vi "CompRun.vi"(0 "Initial Soak":T1(ring)=enum."5 mins", 1 "Nominal":dbl=1.0 min=0.0 max=1000.0 format="%.4f", 2 "Frequency Channel":enum16{"Channel 1", "Channel 2", "Channel 3"}(ring), 3 "Tolerence":dbl=0.01 min=0.001 max=100.0 format="%.2f", 4 "Dmm Readings":i8=5 min=0 max=5 step=1, 5 "Step Soak":T1(ring)=enum."5 mins", 6 "Gate Time":T2(ring)=enum."1.0 second", 7 "HP Switcher Address":cluster{"GPIB":u8, "Address":u8}={"GPIB"=1, "Address"=6} {"Address" min=1 max=31; "GPIB" min=1 max=5}, 8 "Temperature Array":dbl[](array[numeric]), 9 "Final Soak":T1(ring)=enum."5 mins", 11 "Slew Rate":enum16{"0.5", "1", "2"}(ring)=enum."1", 12 "V inj Min":dbl min=0.0 max=20.0 format="%.4f", 14 "Vinj Max":dbl=6.0 min=-6.0 max=20.0 format="%.4f", 15 "Chamber Address":cluster{"GPIB #":u8, "Address":u8}={"GPIB #"=0, "Address"=28}) -> ()   [LabVIEW 2024]
panel:
  out "Output File":path
  in  "DC_SN(s)":string[](array[string])
  in  "WorkOrder":string
  in  "NumberOfUnits":i32
  in  "Output Terminals(+6 V:0)":u16(ring) items=["+6 V output", "+25 V output", "-25 V output"]
  in  "Frequency Counter Address":i16=3 max=31
  out "Measured Frequency":dbl[](array[numeric]) format="%.6f"
  out "Pullability":dbl[](array[numeric]) format="%.6f"
  out "Error":dbl[](array[numeric]) format="%.2f"
  out "Iteration Successful":bool[](array[boolean])
  out "V_inject":dbl[](array[numeric]) format="%.6f"
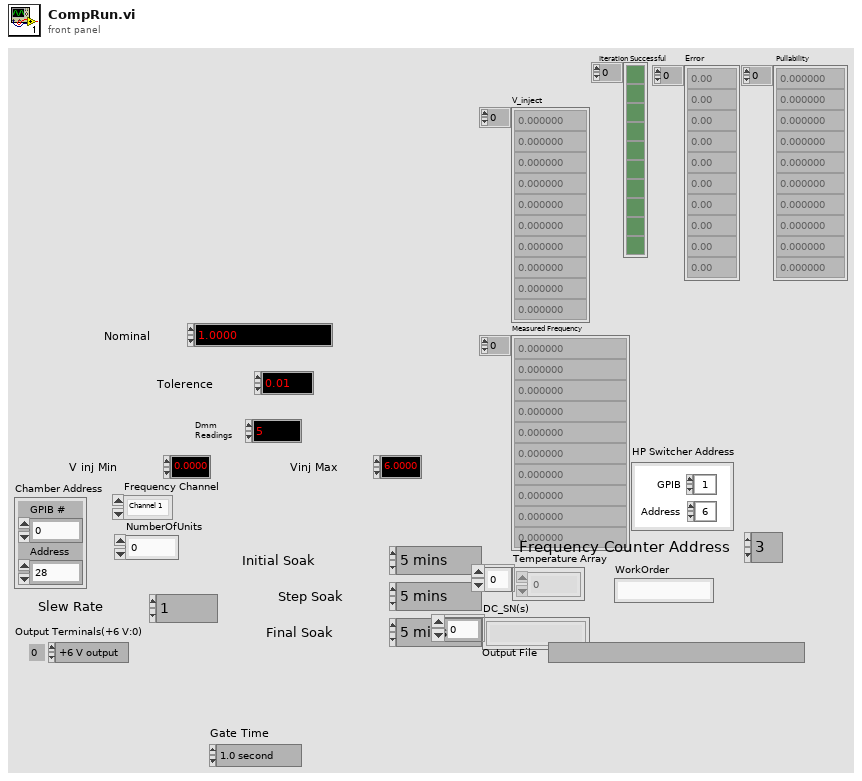
[diagram p1: front panel]
types:
  T1 = enum16{"1 min", "5 mins", "10 mins", "20 mins", "30 mins", "40 mins", "50 mins", "1 hour", "2 hours", "3 hours"}
  T2 = enum16{"0.1 second", "1.0 second", "10.0 second"}
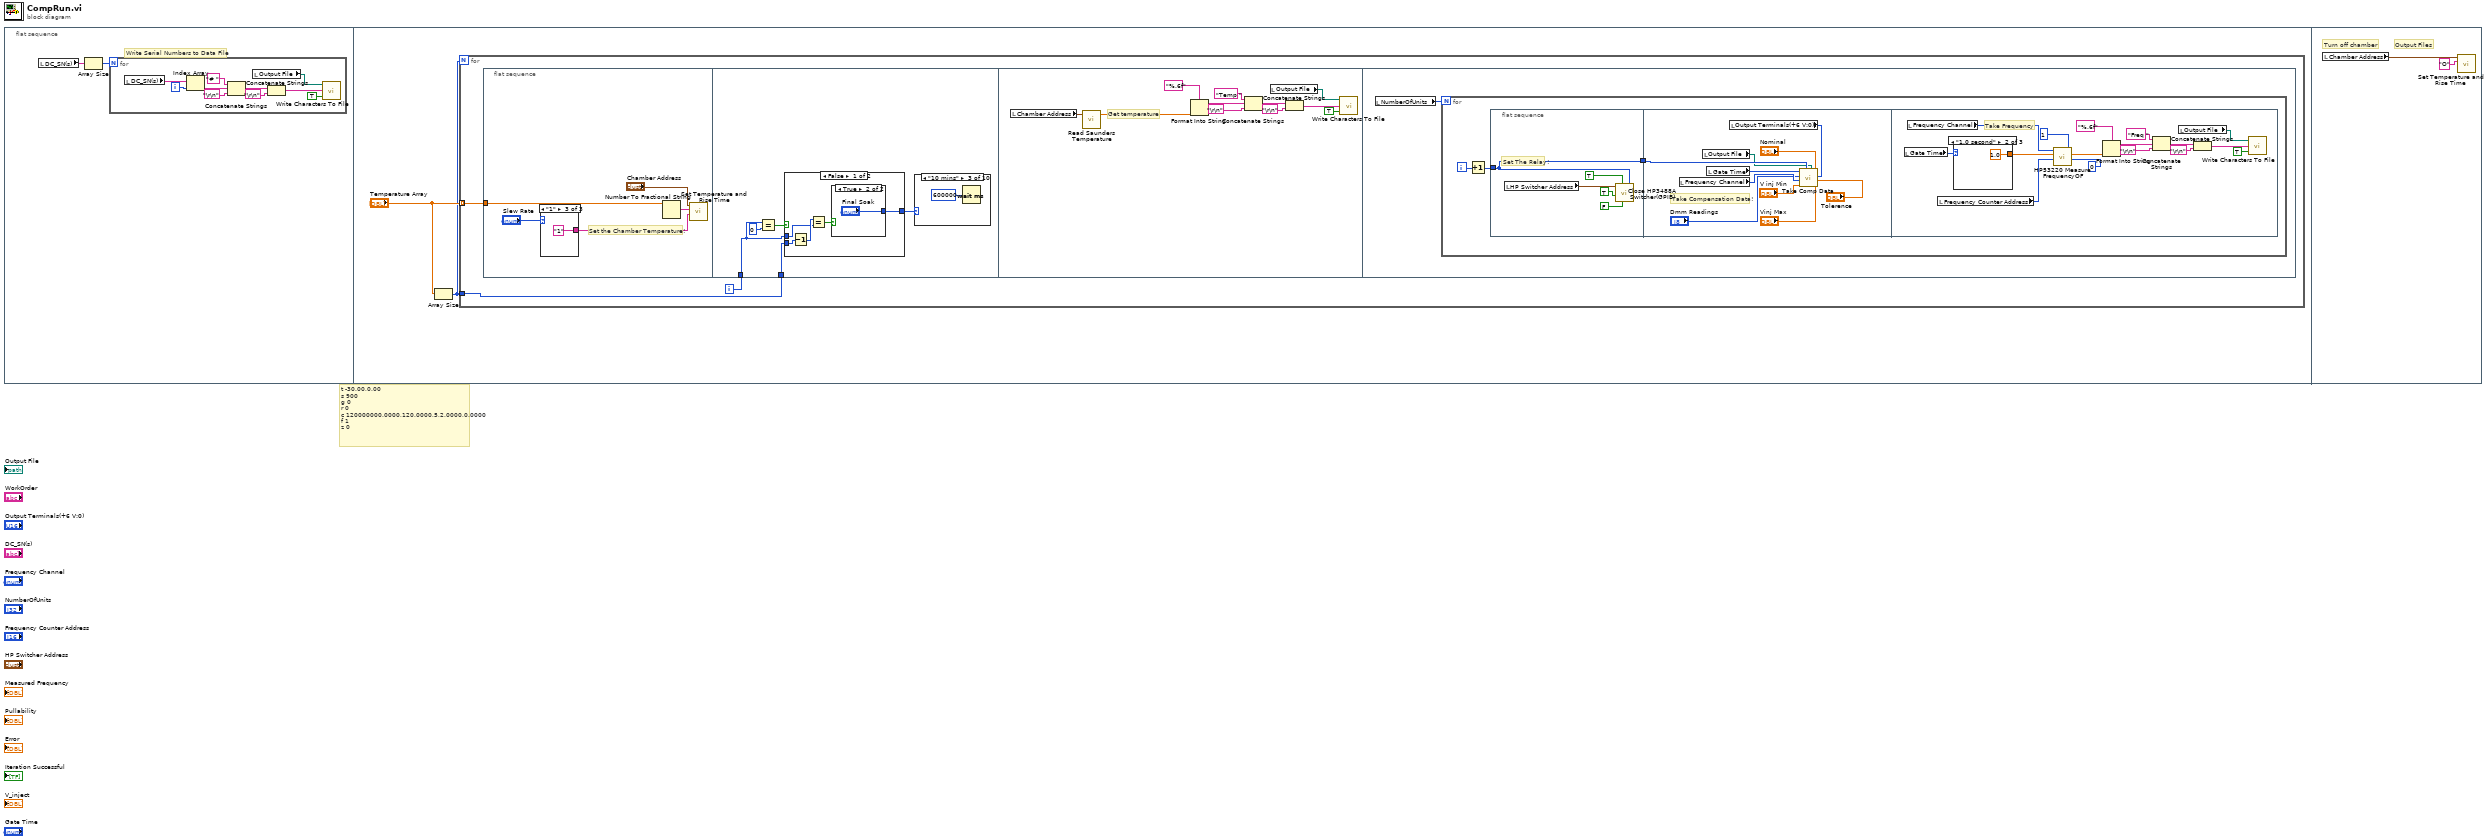
[diagram p0: block diagram]
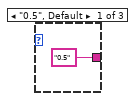
[diagram p2: hidden frame]
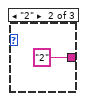
[diagram p3: hidden frame]
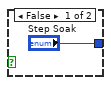
[diagram p4: hidden frame]
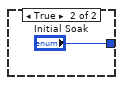
[diagram p5: hidden frame]
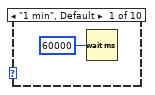
[diagram p6: hidden frame]
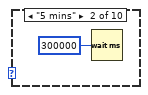
[diagram p7: hidden frame]
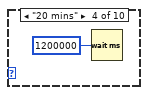
[diagram p8: hidden frame]
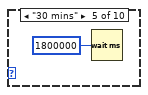
[diagram p9: hidden frame]
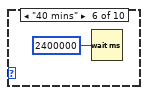
[diagram p10: hidden frame]
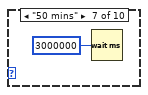
[diagram p11: hidden frame]
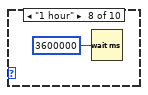
[diagram p12: hidden frame]
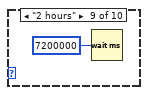
[diagram p13: hidden frame]
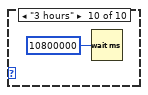
[diagram p14: hidden frame]
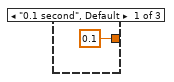
[diagram p15: hidden frame]
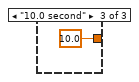
[diagram p16: hidden frame]
diagram:
  # "t -30.00,0.00\ns 900\ng 0\nr 0\nc 120000000.0000,120.0000,5,2.0000,0.0000\nf 1\nz 0"
  n1 = flat-sequence {
    frame #0 {
      # "Write Serial Numbers to Data File"
      n2 = local read "DC_SN(s)"() -> (w1:string[])
      n3 = Array Size(array=w1) -> (size(s)=w2:i32)
      n4 = for {
        N: w2 -> [_]
        i -> [w11]
        n5 = local read "DC_SN(s)"() -> (w12:string[])
        n6 = Index Array(array=w12, index=w11) -> (element=w4:string)
        n7 = Concatenate Strings("# " ("Substring"), w4, "\r\n") -> (w9:string)
        n8 = local read "Output File"() -> (w10:path)
        n9 = Concatenate Strings(w9, "\r\n") -> (w8:string)
        n10 = call "Write Characters To File.vi"("append to file? (new file:F)"=TRUE, "character string"=w8, "file path (dialog if empty)"=w10) -> ()  [unwired: 2 in, 1 out]
      }
    }
    frame #1 {
      n11 = Array Size(array="Temperature Array") -> (size(s)=w13:i32)
      n12 = for {
        N: w13 -> [_]
        tunnel: "Temperature Array" -> [w17] mode=indexing
        tunnel: w13 -> [w16]
        i -> [w15]
        n13 = flat-sequence {
          tunnel: w17 -> [w18]
          tunnel: w16 -> [w28]
          tunnel: w15 -> [w26]
          frame #0 {
            # "Set the Chamber Temperature!"
            n14 = case shown="\"1\"" "Slew Rate" {
              tunnel: ["0.5" ("string") "2" ("string") "1" ("string")] -> w21
              frame "0.5", Default {
              }
              frame "2" {
              }
              frame "1" {
              }
            }
            n15 = Number To Fractional String(number=w18) -> (F-format string=w22:string)  [unwired: 3 in]
            n16 = call "Set Temperature and Rise Time.vi"("Slew Time String"=w21, "Temperature String"=w22, "Device"="Chamber Address") -> ()  [unwired: 3 in, 1 out]
          }
          frame #1 {
            n17 = Equal?(x=w26, y=0) -> (x = y?=w27:bool)
            n18 = case shown="False" w27 {
              tunnel: [w35 "Initial Soak"] -> w29
              tunnel: w28 -> [w33 _]
              tunnel: w26 -> [w31 _]
              frame False {
                n19 = Decrement(x=w33) -> (x-1=w32:i32)
                n20 = Equal?(x=w32, y=w31) -> (x = y?=w34:bool)
                n21 = case shown="True" w34 {
                  tunnel: ["Step Soak" "Final Soak"] -> w35
                  frame False {
                  }
                  frame True {
                  }
                }
              }
              frame True {
              }
            }
            n22 = case shown="\"10 mins\"" w29 {
              frame "1 min", Default {
                n23 = Wait (ms)(milliseconds to wait=u32 60000) -> ()  [unwired: 1 out]
              }
              frame "5 mins" {
                n24 = Wait (ms)(milliseconds to wait=u32 300000) -> ()  [unwired: 1 out]
              }
              frame "10 mins" {
                n25 = Wait (ms)(milliseconds to wait=u32 600000) -> ()  [unwired: 1 out]
              }
              frame "20 mins" {
                n26 = Wait (ms)(milliseconds to wait=u32 1200000) -> ()  [unwired: 1 out]
              }
              frame "30 mins" {
                n27 = Wait (ms)(milliseconds to wait=u32 1800000) -> ()  [unwired: 1 out]
              }
              frame "40 mins" {
                n28 = Wait (ms)(milliseconds to wait=u32 2400000) -> ()  [unwired: 1 out]
              }
              frame "50 mins" {
                n29 = Wait (ms)(milliseconds to wait=u32 3000000) -> ()  [unwired: 1 out]
              }
              frame "1 hour" {
                n30 = Wait (ms)(milliseconds to wait=u32 3600000) -> ()  [unwired: 1 out]
              }
              frame "2 hours" {
                n31 = Wait (ms)(milliseconds to wait=u32 7200000) -> ()  [unwired: 1 out]
              }
              frame "3 hours" {
                n32 = Wait (ms)(milliseconds to wait=u32 10800000) -> ()  [unwired: 1 out]
              }
            }
          }
          frame #2 {
            # "Get temperature"
            n33 = local read "Chamber Address"() -> (w59:cluster{"GPIB #":u8, "Address":u8})
            n34 = call "Read Saunders Temperature.vi"("Device"=w59) -> ("Temperature"=w54:dbl)  [unwired: 3 in, 1 out]
            n35 = Format Into String(format string="%.6f" ("Format String"), w54) -> (resulting string=w58:string)  [unwired: 2 in, 1 out]
            n36 = Concatenate Strings("Temp " ("Substring"), w58, "\r\n") -> (w56:string)
            n37 = local read "Output File"() -> (w55:path)
            n38 = Concatenate Strings(w56, "\r\n") -> (w57:string)
            n39 = call "Write Characters To File.vi"("append to file? (new file:F)"=TRUE, "character string"=w57, "file path (dialog if empty)"=w55) -> ()  [unwired: 2 in, 1 out]
          }
          frame #3 {
            n40 = local read "NumberOfUnits"() -> (w60:i32)
            n41 = for {
              N: w60 -> [_]
              i -> [w62]
              n42 = Increment(x=w62) -> (x+1=w63:i32)
              n43 = flat-sequence {
                tunnel: w63 -> [w64]
                tunnel: [w64] -> w61
                tunnel: w61 -> [w70]
                frame #0 {
                  # "Set The Relay!"
                  n44 = local read "HP Switcher Address"() -> (w68:cluster{"GPIB":u8, "Address":u8})
                  n45 = call "Close HP3488A Switcher(GPIB).vi"("Device In"=w68, "reset"=TRUE, "Use Card# 5"=TRUE, "ID query"=FALSE, "Position Number"=w64) -> ()  [unwired: 3 in, 1 out]
                }
                frame #1 {
                  # "Take Compensation Data!"
                  n46 = local read "Frequency Channel"() -> (w73:enum16{"Channel 1", "Channel 2", "Channel 3"})
                  n47 = local read "Output File"() -> (w69:path)
                  n48 = local read "Gate Time"() -> (w72:T2)
                  n49 = local read "Output Terminals(+6 V:0)"() -> (w71:u16)
                  n50 = call "Take Comp Data.vi"("Maximum V_Inject"="Vinj Max", "Tolerence"="Tolerence", "Output Terminals(+6 V:0)"=w71, "Nominal Frequency"="Nominal", "Output File"=w69, "Oscillator Under Test"=w70, "Minimum V_Inject"="V inj Min", "Dmm Readings"="Dmm Readings", "Frequency Channel"=w73, "Gate Time"=w72) -> ()  [unwired: 1 in]
                }
                frame #2 {
                  # "Take Frequency"
                  n51 = local read "Gate Time"() -> (w94:T2)
                  n52 = local read "Frequency Channel"() -> (w89:enum16{"Channel 1", "Channel 2", "Channel 3"})
                  n53 = local read "Frequency Counter Address"() -> (w92:i16)
                  n54 = case shown="\"1.0 second\"" w94 {
                    tunnel: [0.1 ("Gate Time") 1.0 ("Gate Time") 10.0 ("Gate Time")] -> w93
                    frame "0.1 second", Default {
                    }
                    frame "1.0 second" {
                    }
                    frame "10.0 second" {
                    }
                  }
                  n55 = call "HP53220 Measure FrequencyOF.vi"("GPIB Bus"=0, "Number of Readings"=1, "GPIB Address"=w92, "Gate Time"=w93, "Channel(1,2,3)"=w89) -> ("Frequency"=w80:dbl)  [unwired: 1 in, 1 out]
                  n56 = Format Into String(format string="%.6f" ("Format String"), w80) -> (resulting string=w86:string)  [unwired: 2 in, 1 out]
                  n57 = Concatenate Strings("Freq " ("Substring"), w86, "\r\n") -> (w81:string)
                  n58 = local read "Output File"() -> (w79:path)
                  n59 = Concatenate Strings(w81, "\r\n") -> (w84:string)
                  n60 = call "Write Characters To File.vi"("append to file? (new file:F)"=TRUE, "character string"=w84, "file path (dialog if empty)"=w79) -> ()  [unwired: 2 in, 1 out]
                }
              }
            }
          }
        }
      }
    }
    frame #2 {
      # "Turn off chamber"
      # "Output Files"
      n61 = local read "Chamber Address"() -> (w99:cluster{"GPIB #":u8, "Address":u8})
      n62 = call "Set Temperature and Rise Time.vi"("Temperature String"="O", "Device"=w99) -> ()  [unwired: 4 in, 1 out]
    }
  }
